vi "Priority Benchmark Project.vi"() -> ()   [LabVIEW 2020]
doc: "This example gathers timing information about a VI's execution by running the VI over several iterations. The example obtains several consecutive timestamps, which are stored in an array and used to produce a histogram of execution time. The example can self-calibrate by subtracting out the overhead of calling NI Get Timestamp.vi from the array of timing data."
uses:
  <vilib>/Platform/TimedLoop/XDataNode/timing_clust.ctl
  <vilib>/Platform/TimedLoop/XDataNode/nitl_modes.ctl
  <vilib>/Platform/TimedLoop/XDataNode/wakeup.ctl
  <vilib>/Analysis/Matrix/Numeric/Conversions/Array To Matrix - RA.vi
  <vilib>/Analysis/Matrix/Numeric/Conversions/Array To Matrix - RA2.vi
  <vilib>/Analysis/Matrix/Numeric/Multiply/Multiply - RM,RM.vi
  <vilib>/platform/TimedLoop/XDataNode/XDataNode.xnode
  <vilib>/NI_Real-Time Target Support.lvlib
  <vilib>/Analysis/Matrix/NI_Matrix.lvlib
  <vilib>/Platform/TimedLoop/XDataNode/XDNodeRunTimeDep.lvlib
panel:
  in  "vector size":i32=20
  out "Mean time (us)":dbl format="%.3g"
  out "Max jitter (us)":dbl format="%.3g"
  out "Standard deviation (us)":dbl format="%.3g"
  in  "Warmup iterations":i32=10
  in  "Calibrate?":bool
  in  "Iterations":i32=1000
  out "Execution histogram":T1(graph)
  out "Execution times (us)":dbl[](graph)
  # "Overview: Gathers timing information on VI execution by running it over several iterations.\nRequirements: LabVIEW Real-Time Module\nInstructions:\n1. In Measurement & Automation Explorer, ensure that LabVIEW Real-Time is installed on your RT target.  \n2. From the Project Explorer window, set the IP address of your RT target.\n3. From the front panel, select the number of iterations to run and the number of warmup iterations to exclude from the benchmark.\n4. Enable Calibrate? if you want to exclude the overhead of the timestamping operation.\n5. Open the block diagram and insert the code you want to benchmark in the #CodeNeeded section.\n6. Run the VI."
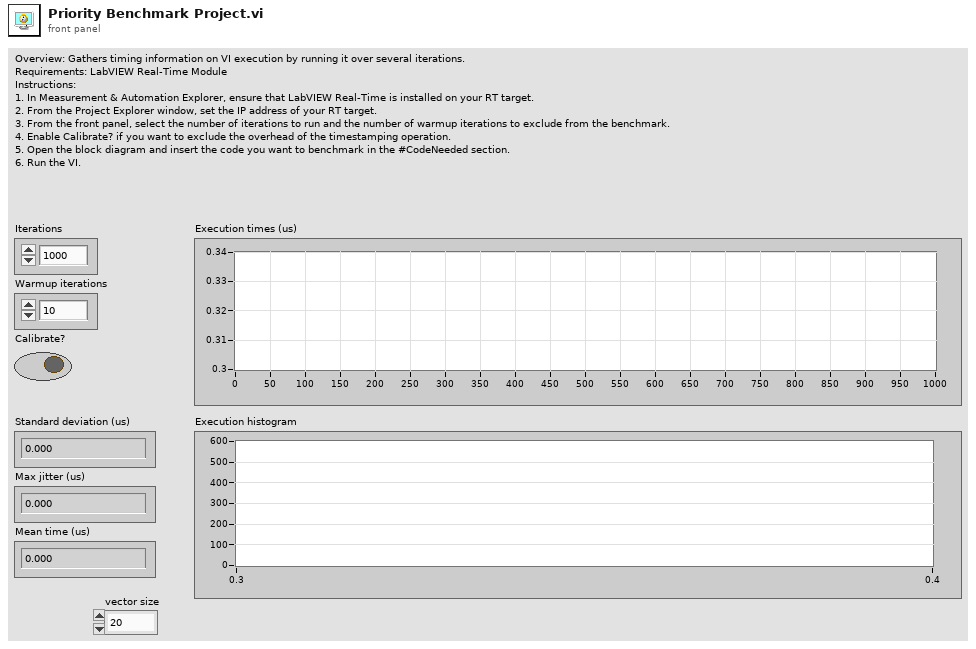
[diagram p1: front panel]
types:
  T1 = cluster{"X Values":dbl[], "Histogram: h(x)":i32[]}
  T2 = typedef "XDNodeRunTimeDep.lvlib/timing_clust.ctl" = cluster{"Expected End [f-1]":u64, "Actual End [f-1]":u64, "Finished Late? [f-1]":bool, "Expected End [i-1]":u64, "Actual End [i-1]":u64, "Finished Late? [i-1]":bool, "Expected Start [i]":u64, "Actual Start [i]":u64, "Expected Start [f]":u64, "Actual Start [f]":u64, "Source Name":string, "Structure Name":string, "Period":i64, "Deadline":i64, "Offset":i64, "Start":i64, "Priority":i32, "Timeout":i32, "Mode":T3, "Wakeup Reason":T4, "Error":errorcluster, "Source Type":string, "Secondary Source Type":string, "Global End Time":u64, "Global Start Time":u64, "Frame Duration":u64, "Iteration Duration":u64, "Assigned CPU":i32, "I/O Scan Engine Mode":u32}
  T3 = typedef "XDNodeRunTimeDep.lvlib/nitl_modes.ctl" = enum32{"No Change", "Process missed periods, maintain original phase", "Discard missed periods, maintain original phase", "Process missed periods, ignore original phase", "Discard missed periods, ignore original phase"}
  T4 = typedef "XDNodeRunTimeDep.lvlib/wakeup.ctl" = enum32{"Normal", "Aborted", "Asynchronous wakeup", "Timing source error", "Timed loop error", "Timeout"}
  T5 = typedef "NI_Matrix.lvlib/RealMatrix.ctl" = dbl[][]
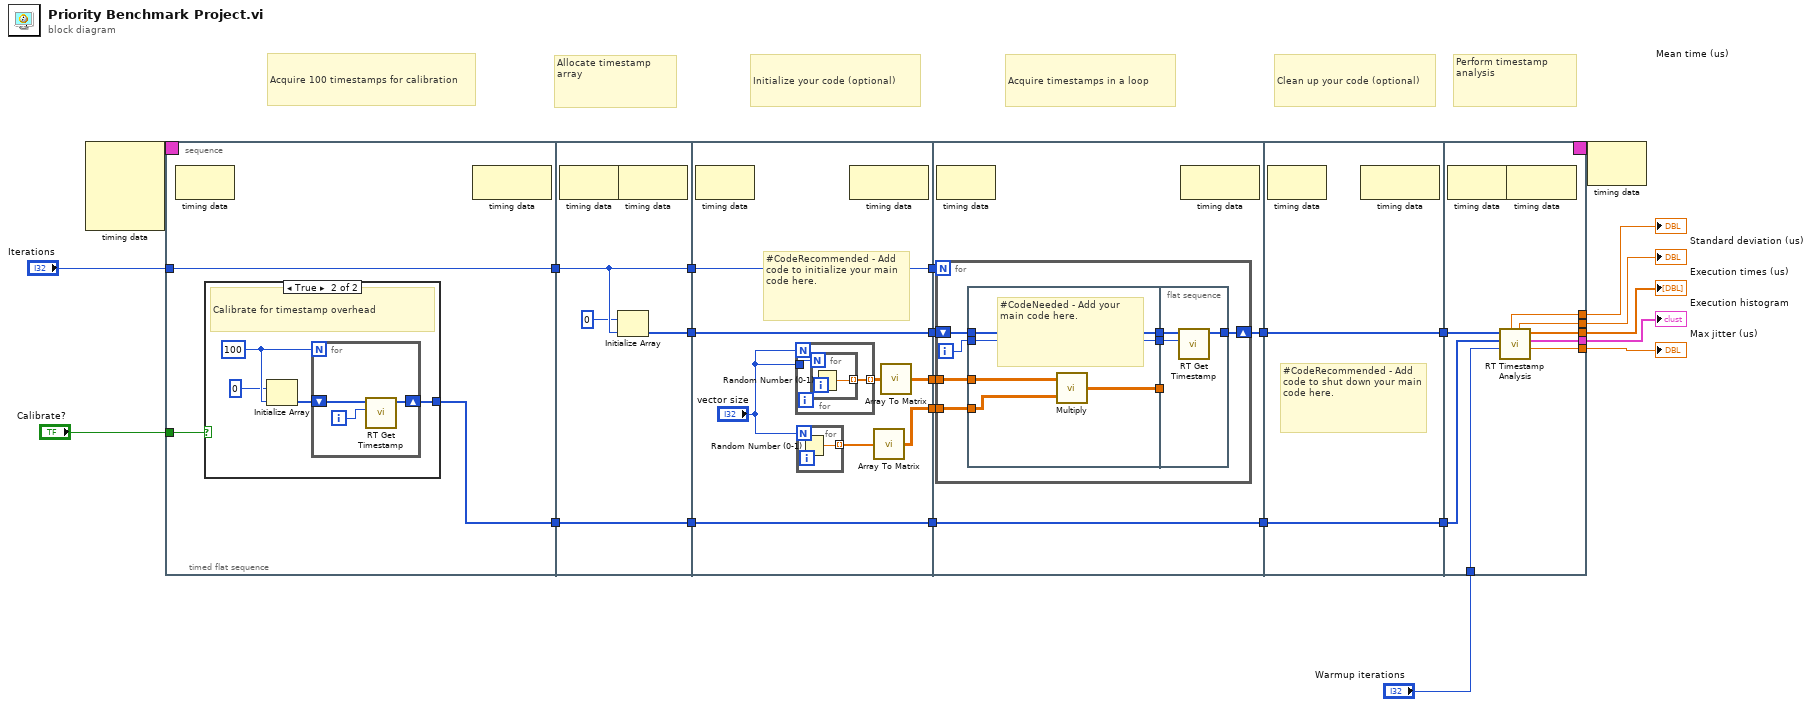
[diagram p0: block diagram]
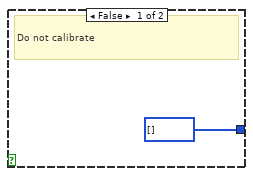
[diagram p2: hidden frame]
diagram:
  # "Perform timestamp analysis"
  # "Clean up your code (optional)"
  # "Acquire timestamps in a loop"
  # "Initialize your code (optional)"
  # "Allocate timestamp array"
  # "Acquire 100 timestamps for calibration"
  n1 = node-c288() -> (w2:T2)  [unwired: 4 in]
  n2 = timed-sequence {
    timing: w2 -> [_]
    timing-out: [_] -> w1
    tunnel: "Iterations" -> [w32]
    tunnel: "Calibrate?" -> [w31]
    tunnel: [w21] -> w3
    tunnel: [w20] -> w7
    tunnel: [w19] -> w6
    tunnel: [w18] -> w8
    tunnel: "Warmup iterations" -> [w17]
    tunnel: [w16] -> w4
    n3 = timed-flat-sequence {
      tunnel: w32 -> [w35]
      tunnel: [w35] -> w30
      tunnel: w31 -> [w34]
      tunnel: [w33] -> w11
      tunnel: [w48] -> w29
      tunnel: [w49] -> w28
      tunnel: w30 -> [w48]
      tunnel: [w46] -> w12
      tunnel: w11 -> [w46]
      tunnel: [w59] -> w27
      tunnel: [w58] -> w26
      tunnel: w29 -> [w59]
      tunnel: w28 -> [w58]
      tunnel: [w54] -> w25
      tunnel: [w53] -> w24
      tunnel: [w52] -> w13
      tunnel: w12 -> [w52]
      tunnel: [w71] -> w23
      tunnel: w27 -> [w70]
      tunnel: w26 -> [w69]
      tunnel: w25 -> [w68]
      tunnel: w24 -> [w67]
      tunnel: [w66] -> w14
      tunnel: w13 -> [w66]
      tunnel: w23 -> [w91]
      tunnel: [w91] -> w22
      tunnel: [w90] -> w15
      tunnel: w14 -> [w90]
      tunnel: w22 -> [w101]
      tunnel: [w100] -> w21
      tunnel: [w99] -> w20
      tunnel: [w98] -> w19
      tunnel: [w97] -> w18
      tunnel: w17 -> [w96]
      tunnel: [w95] -> w16
      tunnel: w15 -> [w94]
      frame #0 {
        n4 = node-c288() -> ()  [unwired: 1 in, 1 out]
        n5 = case shown="True" w34 {
          tunnel: [u64[] [] w42] -> w33
          frame False {
            # "Do not calibrate"
          }
          frame True {
            w40 = 100
            # "Calibrate for timestamp overhead"
            n6 = Initialize Array(u64 0, w40) -> (w41:u64[])
            n7 = for {
              N: w40 -> [_]
              shift-right: [w43] -> w42
              shift-left: w41 -> [w44]
              i -> [w45]
              n8 = call <vilib>:"RT Get Timestamp.vi"("iteration"=w45, "timestamp array in"=w44) -> ("timestamp array out"=w43:u64[])  [unwired: 1 in, 8 out]
            }
          }
        }
        n9 = node-c288() -> ()  [unwired: 1 in, 1 out]
      }
      frame #1 {
        n10 = node-c288() -> ()  [unwired: 1 in, 1 out]
        n11 = node-c288() -> ()  [unwired: 1 in, 1 out]
        n12 = Initialize Array(u64 0, w48) -> (w49:u64[])
      }
      frame #2 {
        # "#CodeRecommended - Add code to initialize your main code here."
        n13 = node-c288() -> ()  [unwired: 1 in, 1 out]
        n14 = for {
          N: "vector size" -> [_]
          tunnel: [w63] -> w56 mode=indexing
          tunnel: "vector size" -> [w62]
          n15 = for {
            N: w62 -> [_]
            tunnel: [w64] -> w63 mode=indexing
            n16 = Random Number (0-1)() -> (number: 0 to 1=w64:dbl)
          }
        }
        n17 = for {
          N: "vector size" -> [_]
          tunnel: [w65] -> w57 mode=indexing
          n18 = Random Number (0-1)() -> (number: 0 to 1=w65:dbl)
        }
        n19 = node-c288() -> ()  [unwired: 1 in, 1 out]
        n20 = call-poly <vilib>:"Array To Matrix.vi"("Real 1D Array"=w57) -> ("Real Matrix (Column Vector)"=w53:T5)
        n21 = call-poly <vilib>:"Array To Matrix.vi"("Real 2D Array"=w56) -> ("Real Matrix"=w54:T5)
      }
      frame #3 {
        n22 = for {
          N: w70 -> [_]
          shift-right: [w81] -> w71
          shift-left: w69 -> [w80]
          tunnel: w68 -> [w76]
          tunnel: w67 -> [w75]
          i -> [w79]
          n23 = flat-sequence {
            tunnel: w80 -> [w86]
            tunnel: [w86] -> w78
            tunnel: w79 -> [w85]
            tunnel: [w85] -> w77
            tunnel: w76 -> [w84]
            tunnel: w75 -> [w83]
            tunnel: [w82] -> w74
            tunnel: [w89] -> w81
            tunnel: w78 -> [w87]
            tunnel: w77 -> [w88]
            tunnel: w74 -> [_]
            frame #0 {
              # "#CodeNeeded - Add your main code here."
              n24 = call-poly <vilib>:"Multiply.vi"("Real Matrix B"=w83, "Real Matrix A"=w84) -> ("A * B"=w82:T5)
            }
            frame #1 {
              n25 = call <vilib>:"RT Get Timestamp.vi"("iteration"=w88, "timestamp array in"=w87) -> ("timestamp array out"=w89:u64[])  [unwired: 1 in, 8 out]
            }
          }
        }
        n26 = node-c288() -> ()  [unwired: 1 in, 1 out]
        n27 = node-c288() -> ()  [unwired: 1 in, 1 out]
      }
      frame #4 {
        # "#CodeRecommended - Add code to shut down your main code here."
        n28 = node-c288() -> ()  [unwired: 1 in, 1 out]
        n29 = node-c288() -> ()  [unwired: 1 in, 1 out]
      }
      frame #5 {
        n30 = node-c288() -> ()  [unwired: 1 in, 1 out]
        n31 = node-c288() -> ()  [unwired: 1 in, 1 out]
        n32 = call <vilib>:"RT Timestamp Analysis.vi"("warmup iterations"=w96, "calibration array"=w94, "timestamp array"=w101) -> ("max jitter (uS)"=w99:dbl, "execution histogram"=w100:T1, "execution times (uS)"=w97:dbl[], "standard deviation (uS)"=w98:dbl, "mean time (uS)"=w95:dbl)  [unwired: 1 in, 3 out]
      }
    }
  }
  "Execution times (us)" <- w8
  "Max jitter (us)" <- w7
  "Standard deviation (us)" <- w6
  "Execution histogram" <- w3
  "Mean time (us)" <- w4
  n33 = node-c288(w1) -> ()  [unwired: 1 out]
